vi "Queue Command Bundle.vi"(10 "Variant Data":variant, 11 "Command":string) -> (3 "main window queue datatype":T1)   [LabVIEW 2018]
doc: "Bundles Command String and anything else into the variant as Argument. Outputs Command Q cluster.\n\n2007 Mike Ashe\nmichael.ashe@imaginatics.net\nCell: 860-961-0876"
uses:
  Command Queue Cluster.ctl
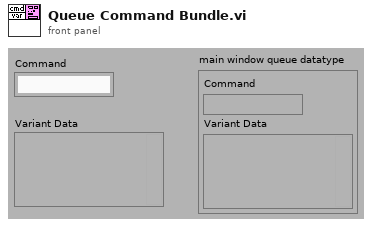
[diagram p1: front panel]
types:
  T1 = typedef "Command Queue Cluster.ctl" = cluster{"Command":string, "Variant Data":variant}
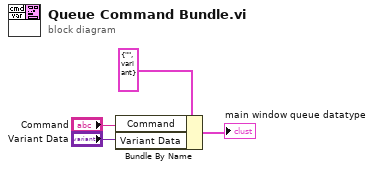
[diagram p0: block diagram]
diagram:
  n1 = Bundle By Name(cluster=T1 {"Command"="", "Variant Data"=variant} ("queue data"), "Command"="Command", "Variant Data"="Variant Data") -> (→"main window queue datatype":T1)
